vi "From Variant.vi"(0 "Obj in":refnum<class "Noise.lvclass">, 7 "Variant":variant, 9 "Prefix":string, 11 "error in (no error)":errorcluster) -> (4 "Obj out":refnum<class "Noise.lvclass">, 15 "error out":errorcluster)   [LabVIEW 2020, in "Noise.lvclass"]
uses:
  Noise.lvclass
  Noise.lvclass/Noise.ctl
  Waveform/Waveform.lvclass
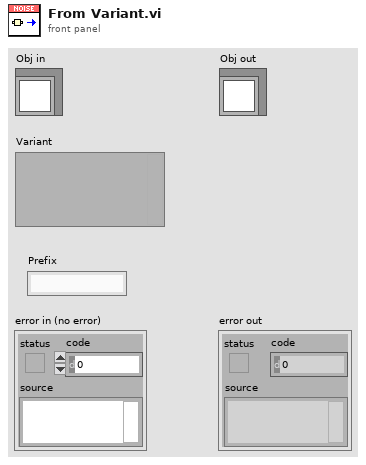
[diagram p1: front panel]
types:
  T1 = typedef "Noise.lvclass/Serialized.ctl" = cluster{"Seed":i32, "Tokens":i32, "InvFilt":bool, "Aweight":bool, "Weights":T2}
  T2 = typedef "Noise.lvclass/Weighting.ctl" = enum16{"White", "Pink"}
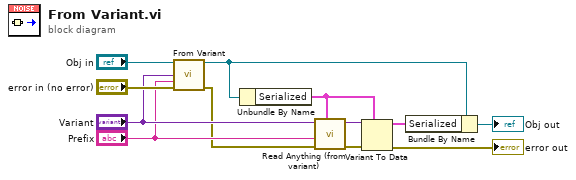
[diagram p0: block diagram]
diagram:
  n1 = call-parent "From Variant.vi"("Obj in"="Obj in", "Variant"="Variant", "Prefix"="Prefix", "error in (no error)"="error in (no error)") -> ("Obj out"=w3:refnum<class "Noise.lvclass">, "error out"=w4:errorcluster)  [unwired: 10 in]
  n2 = Unbundle By Name(w3) -> ("Serialized"=w8:T1)
  n3 = call "Read Anything (from variant).vi"("Type of Anything"=w8, "Error In"=w4, "Prefix"="Prefix", "Variant Database"="Variant") -> ("Error Out"=w9:errorcluster, "Anything"=w10:variant)  [unwired: 5 in, 1 out]
  n4 = Variant To Data(error in=w9, type=w8, Variant=w10) -> (data=w7:T1, error out=→"error out":errorcluster)
  n5 = Bundle By Name(cluster=w3, "Serialized"=w7) -> (→"Obj out":refnum<class "Noise.lvclass">)
